vi "Restore Scale Property.vi"(4 "Control Ref Cluster":T1, 6 "Update?":bool=TRUE, 7 "Polor?":bool, 8 "error in (no error)":errorcluster, 11 "2D Plot.lvclass in":refnum<class "2D Plot.lvclass">) -> (0 "error out":errorcluster, 3 "2D Plot.lvclass out":refnum<class "2D Plot.lvclass">)   [LabVIEW 2020, in "2D Plot.lvclass"]
uses:
  <vilib>/Math Plots/2D Math Plots/2D Plot/2D Plot/2D Plot.lvclass
  <vilib>/Math Plots/2D Math Plots/2D Plot/Action String/2DMathPlot Ctrl Act Cluster.ctl
  <vilib>/Math Plots/2D Math Plots/2D Plot/Action String/2DMathPlot State Class.ctl
  <vilib>/Math Plots/2D Math Plots/2D Plot/2D Plot/2D Plot.lvclass/2D Plot.ctl
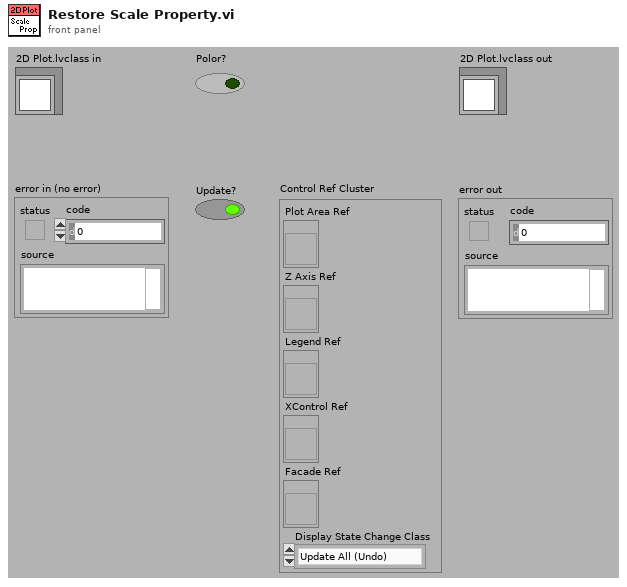
[diagram p1: front panel]
types:
  T1 = typedef "2DMathPlot Ctrl Act Cluster.ctl" = cluster{"Plot Area Ref":refnum<vi>, "Z Axis Ref":refnum<vi>, "Legend Ref":refnum<vi>, "XControl Ref":refnum<vi>, "Facade Ref":refnum<vi>, "Display State Change Class":T2}
  T2 = typedef "2DMathPlot State Class.ctl" = enum16{"Update All (Undo)", "Update General", "Update Appearance", "Update Format", "Update Scale", "Update Marker", "Update Cursor", "None"}
  T3 = typedef "2D Plot.lvclass/Scale Array.ctl" = T4[]
  T4 = typedef "2D Plot.lvclass/Scale Cluster.ctl" = cluster{"General":cluster{"Editable":bool, "Flipped":bool, "Mapping Mode":u8, "Visible":bool, "Style":u8, "Scale Fit":u8}, "Offset and Multiplier":T5, "Range":cluster{"Minimum":dbl, "Maximum":dbl, "Increment":dbl, "Minor Increment":dbl, "Start":dbl}, "Tick Color":cluster{"Major Color":u32, "Minor Color":u32}, "Gird Color":cluster{"Major Color":u32, "Minor Color":u32}, "Marker":cluster{"Visible":bool, "FG Color":u32, "BG Color":u32, "Font Name":string, "Font Size":u32, "Font Bold":bool, "Font Italic":bool, "Font Strikeout":bool, "Font Underline":bool}, "Name Label":cluster{"Visible":bool, "FG Color":u32, "BG Color":u32, "Font Name":string, "Font Size":u32, "Font Bold":bool, "Font Italic":bool, "Font Strikeout":bool, "Font Underline":bool, "Justification":enum16{"Left", "Center", "Right"}, "Text":string}}
  T5 = typedef "LVOffsetAndMultiplierTypeDef.ctl" = cluster{"Offset":dbl, "Multiplier":dbl}
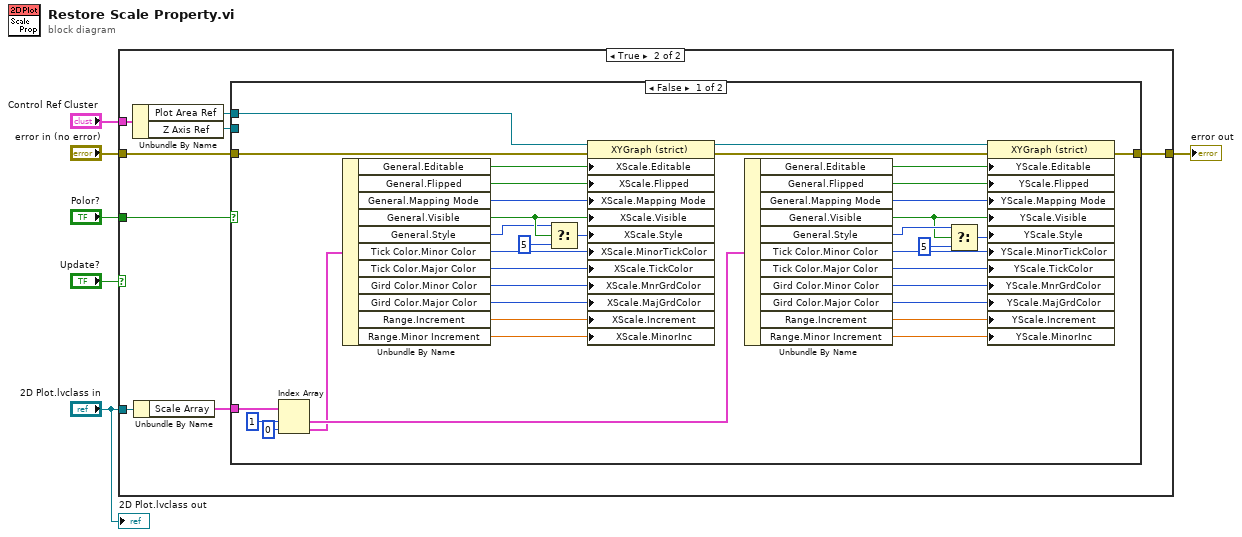
[diagram p0: block diagram]
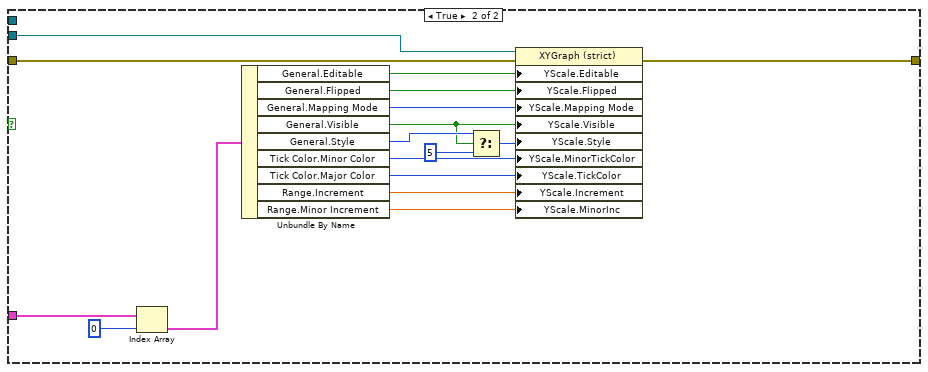
[diagram p3: hidden frame]
diagram:
  n1 = case shown="True" "Update?" {
    tunnel: "2D Plot.lvclass in" -> [_ w15]
    tunnel: "Control Ref Cluster" -> [_ w13]
    tunnel: "Polor?" -> [_ w12]
    tunnel: "error in (no error)" -> [w7 w9]
    tunnel: [w7 w8] -> w2
    frame False {
    }
    frame True {
      n2 = Unbundle By Name(w13) -> ("Plot Area Ref"=w11:refnum<vi>, "Z Axis Ref"=w10:refnum<vi>)
      n3 = Unbundle By Name(w15) -> ("Scale Array"=w14:T3)
      n4 = case shown="False" w12 {
        tunnel: w14 -> [w51 w55]
        tunnel: w11 -> [w50 _]
        tunnel: w10 -> [_ w66]
        tunnel: [w25 w56] -> w8
        tunnel: w9 -> [w41 w64]
        frame False {
          n5 = Index Array(array=w51, index #1=1 ("index"), index #2=0 ("index")) -> (element #1=w46:T4, element #2=w45:T4)
          n6 = Unbundle By Name(w45) -> ("General.Editable"=w37:bool, "General.Flipped"=w49:bool, "General.Mapping Mode"=w48:u8, "General.Visible"=w34:bool, "General.Style"=w33:u8, "Tick Color.Minor Color"=w47:u32, "Tick Color.Major Color"=w20:u32, "Gird Color.Minor Color"=w19:u32, "Gird Color.Major Color"=w18:u32, "Range.Increment"=w24:dbl, "Range.Minor Increment"=w23:dbl)
          n7 = Select(t=w33, s=w34, f=u8 5) -> (s? t:f=w32:u8)
          n8 = property class="XYGraph (strict)"(reference=w50, error in=w41, "XScale.Editable"=w37, "XScale.Flipped"=w49, "XScale.Mapping Mode"=w48, "XScale.Visible"=w34, "XScale.Style"=w32, "XScale.MinorTickColor"=w47, "XScale.TickColor"=w20, "XScale.MnrGrdColor"=w19, "XScale.MajGrdColor"=w18, "XScale.Increment"=w24, "XScale.MinorInc"=w23) -> (reference out=w27:refnum<vi>, error out=w26:errorcluster)
          n9 = Unbundle By Name(w46) -> ("General.Editable"=w36:bool, "General.Flipped"=w44:bool, "General.Mapping Mode"=w43:u8, "General.Visible"=w28:bool, "General.Style"=w30:u8, "Tick Color.Minor Color"=w42:u32, "Tick Color.Major Color"=w40:u32, "Gird Color.Minor Color"=w17:u32, "Gird Color.Major Color"=w16:u32, "Range.Increment"=w22:dbl, "Range.Minor Increment"=w21:dbl)
          n10 = Select(t=w30, s=w28, f=u8 5) -> (s? t:f=w29:u8)
          n11 = property class="XYGraph (strict)"(reference=w27, error in=w26, "YScale.Editable"=w36, "YScale.Flipped"=w44, "YScale.Mapping Mode"=w43, "YScale.Visible"=w28, "YScale.Style"=w29, "YScale.MinorTickColor"=w42, "YScale.TickColor"=w40, "YScale.MnrGrdColor"=w17, "YScale.MajGrdColor"=w16, "YScale.Increment"=w22, "YScale.MinorInc"=w21) -> (error out=w25:errorcluster)  [unwired: 1 out]
        }
        frame True {
          n12 = Index Array(array=w55, index=0) -> (element=w65:T4)
          n13 = Unbundle By Name(w65) -> ("General.Editable"=w61:bool, "General.Flipped"=w68:bool, "General.Mapping Mode"=w67:u8, "General.Visible"=w57:bool, "General.Style"=w58:u8, "Tick Color.Minor Color"=w63:u32, "Tick Color.Major Color"=w62:u32, "Range.Increment"=w54:dbl, "Range.Minor Increment"=w53:dbl)
          n14 = Select(t=w58, s=w57, f=u8 5) -> (s? t:f=w59:u8)
          n15 = property class="XYGraph (strict)"(reference=w66, error in=w64, "YScale.Editable"=w61, "YScale.Flipped"=w68, "YScale.Mapping Mode"=w67, "YScale.Visible"=w57, "YScale.Style"=w59, "YScale.MinorTickColor"=w63, "YScale.TickColor"=w62, "YScale.Increment"=w54, "YScale.MinorInc"=w53) -> (error out=w56:errorcluster)  [unwired: 1 out]
        }
      }
    }
  }
  "error out" <- w2
  "2D Plot.lvclass out" <- "2D Plot.lvclass in"
